vi "FPGA (Top Level) DK.vi"() -> ()   [LabVIEW 2017]
uses:
  <vilib>/LabVIEW Targets/FPGA/cRIO/cRIO-9505/controls.llb/_nicrio_cRIO-9505_DriveStatus.ctl
  <vilib>/Platform/TimedLoop/XDataNode/timing_clust.ctl
  <vilib>/Platform/TimedLoop/XDataNode/nitl_modes.ctl
  <vilib>/Platform/TimedLoop/XDataNode/wakeup.ctl
  <vilib>/rvi/FXPMathLib/FxpSinAndCos/subVIs/nifxpmath_SinAndCos_SimConfig.ctl
  <vilib>/rvi/Emulation/niFpgaGetClockAttributes.vi
  <vilib>/rvi/Emulation/niFpgaSctlEmulationGetInTimedLoop.vi
  <vilib>/rvi/Emulation/niFpgaEmulationReportErrorSimple.vi
  <vilib>/rvi/eio/common/nirviEmuTemplateMethod_errors.vi
  <vilib>/rvi/Emulation/niFpgaEmulationIsFPGAContextNoSignature.vi
  <vilib>/rvi/DataTransferAndStorage/Container/Common/niFpgaContainerGetUniqueNameForEmu.vi
  <vilib>/rvi/Memory/Memory_Emulation/niFpgaMemoryEmulationCacheClearOnFirstRun.vi
  <vilib>/rvi/Memory/Memory_Emulation/nirvimemoryEmulationManagerCache_MakeExclusive.vi
  <vilib>/rvi/Memory/Memory_Emulation/niFpgaMemoryEmulationValidateCache.vi
  <vilib>/rvi/Memory/Memory_Emulation/nirvimemoryEmulationManagerCache_InsertValue.vi
  <vilib>/Utility/error.llb/Clear Errors.vi
  <vilib>/rvi/Memory/Memory_Emulation/nirvimemoryEmulationManagerCache_ReleaseExclusive.vi
  <vilib>/rvi/Memory/Memory_Emulation/nirvimemoryEmulationManagerCache_GetValue.vi
  <vilib>/rvi/Memory/Memory_Emulation/nirvimemoryEmulationManagerCache_SetValue.vi
  <vilib>/rvi/Emulation/niFpgaProcessEmulError.vi
  <vilib>/rvi/Emulation/niFpgaCriticalErrorInLSC.vi
  <vilib>/rvi/FXPMathLib/FxpSinAndCos/simVIs/DllFxpSinAndCosTemp_sub.vi
  <vilib>/eio/EIONode/EIONode.xnode
  <vilib>/rvi/DataTransferAndStorage/Container/XNode/niFpgaContainer.xnode
  <vilib>/rvi/DataTransferAndStorage/Register/Emulation/niFpgaRegisterEmulation.vi
  <vilib>/rvi/FXPMathLib/FxpSinAndCos/XNode/nifxpmath_SinAndCos.xnode
  <vilib>/Platform/TimedLoop/XDataNode/XDataNode.xnode
  <vilib>/Platform/TimedLoop/XDataNode/XDNodeRunTimeDep.lvlib
  <vilib>/eio/EIOMethodNode/EIOMethodNode.xnode
panel:
  in  "Link_1 Duty":i16
  in  "Link_2 Duty":i16
  in  "LINK1_DRIVE_ENABLED":bool
  in  "LINK2_DRIVE_ENABLED":bool
  out "LINK2_DRIVE_STATUS":T1
  out "LINK1_DRIVE_STATUS":T1
  in  "LINK1_LENGTH_MM":fxp<+,16,12>=2.0 format="%#_19g"
  in  "LINK2_LENGTH_MM":fxp<+,16,12>=2.0 format="%#_19g"
  in  "X_OFFSET_MM":fxp<+/-,33,15>
  in  "Y_OFFSET_MM":fxp<+/-,33,15>
  out "LINK2_Y_MM":fxp<+/-,34,16>
  out "LINK2_X_MM":fxp<+/-,34,16>
  out "LINK1_Y_MM":fxp<+/-,34,16>
  out "LINK1_X_MM":fxp<+/-,34,16>
  out "Link 1 Test Y Direction":fxp<+/-,34,16>
  out "LINK1_ENC_POS":i32
  out "LINK2_ENC_POS":i32
  out "LINK1_POT_POS":i32
  out "LINK2_POT_POS":i32
  in  "LINK1_ENC_SCALE":fxp<+,32,0> format="%#_32g"
  in  "LINK2_ENC_SCALE":fxp<+,32,0>=0.029296900611370802 format="%#_32g"
  in  "LINK1_PWM_MAX":i16
  in  "LINK2_PWM_MAX":i16
  in  "LINK1_DEMAND_PWM":i16
  in  "LINK2_DEMAND_PWM":i16
  in  "LINK1_POT_SCALE":fxp<+/-,32,16>
  in  "LINK1_OFFSET":fxp<+/-,16,16>
  in  "LINK2_POT_SCALE":fxp<+/-,32,16>
  in  "LINK2_OFFSET":fxp<+/-,16,16>
  in  "AI_POT_LOOP_US":u16
  in  "ENC_DEBOUNCE_CYCLES":u16=5
  in  "LINK1_ENC_CNTS":i32
  in  "LINK2_ENC_CNTS":i32
  in  "LINK1_UPDATE_ENC":bool
  in  "LINK2_UPDATE_ENC":bool
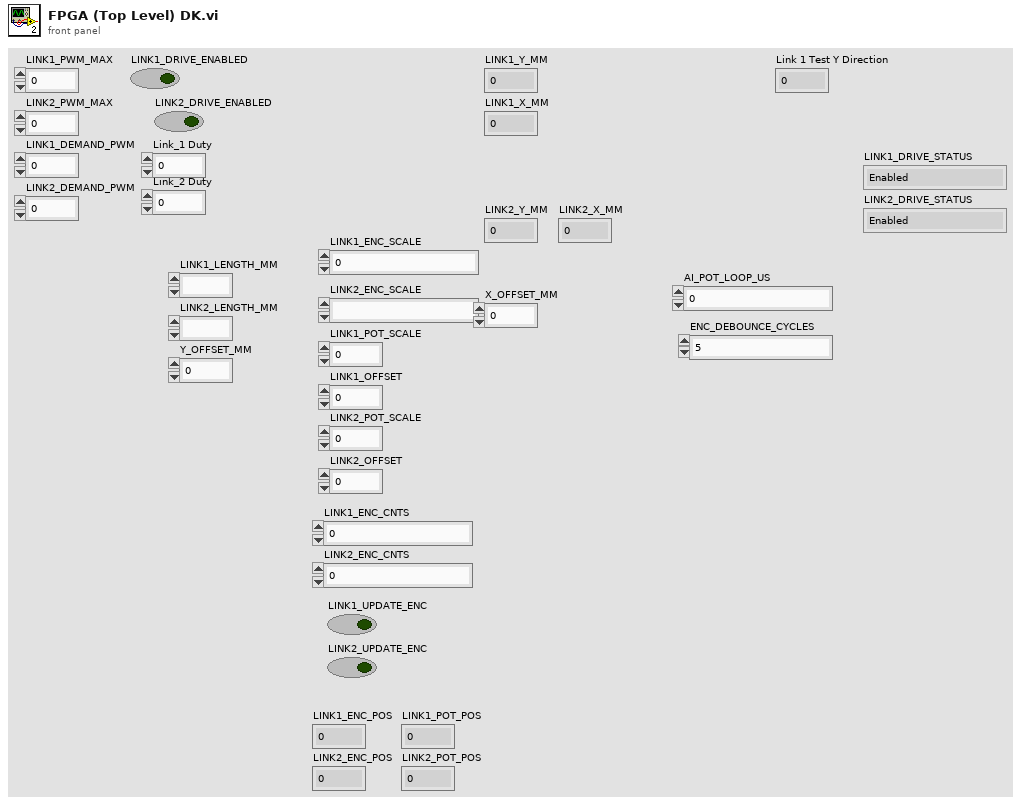
[diagram p1: front panel]
types:
  T1 = typedef "_nicrio_cRIO-9505_DriveStatus.ctl" = enum8{"Enabled", "Disabled", "Disabled by Drive Fault", "Disabled by Temp. Fault", "Disabled by E-Stop", "Unknown"}
  T2 = typedef "XDNodeRunTimeDep.lvlib/timing_clust.ctl" = cluster{"Expected End [f-1]":u64, "Actual End [f-1]":u64, "Finished Late? [f-1]":bool, "Expected End [i-1]":u64, "Actual End [i-1]":u64, "Finished Late? [i-1]":bool, "Expected Start [i]":u64, "Actual Start [i]":u64, "Expected Start [f]":u64, "Actual Start [f]":u64, "Source Name":string, "Structure Name":string, "Period":i64, "Deadline":i64, "Offset":i64, "Start":i64, "Priority":i32, "Timeout":i32, "Mode":T3, "Wakeup Reason":T4, "Error":errorcluster, "Source Type":string, "Secondary Source Type":string, "Global End Time":u64, "Global Start Time":u64, "Frame Duration":u64, "Iteration Duration":u64, "Assigned CPU":i32, "I/O Scan Engine Mode":u32}
  T3 = typedef "XDNodeRunTimeDep.lvlib/nitl_modes.ctl" = enum32{"No Change", "Process missed periods, maintain original phase", "Discard missed periods, maintain original phase", "Process missed periods, ignore original phase", "Discard missed periods, ignore original phase"}
  T4 = typedef "XDNodeRunTimeDep.lvlib/wakeup.ctl" = enum32{"Normal", "Aborted", "Asynchronous wakeup", "Timing source error", "Timed loop error", "Timeout"}
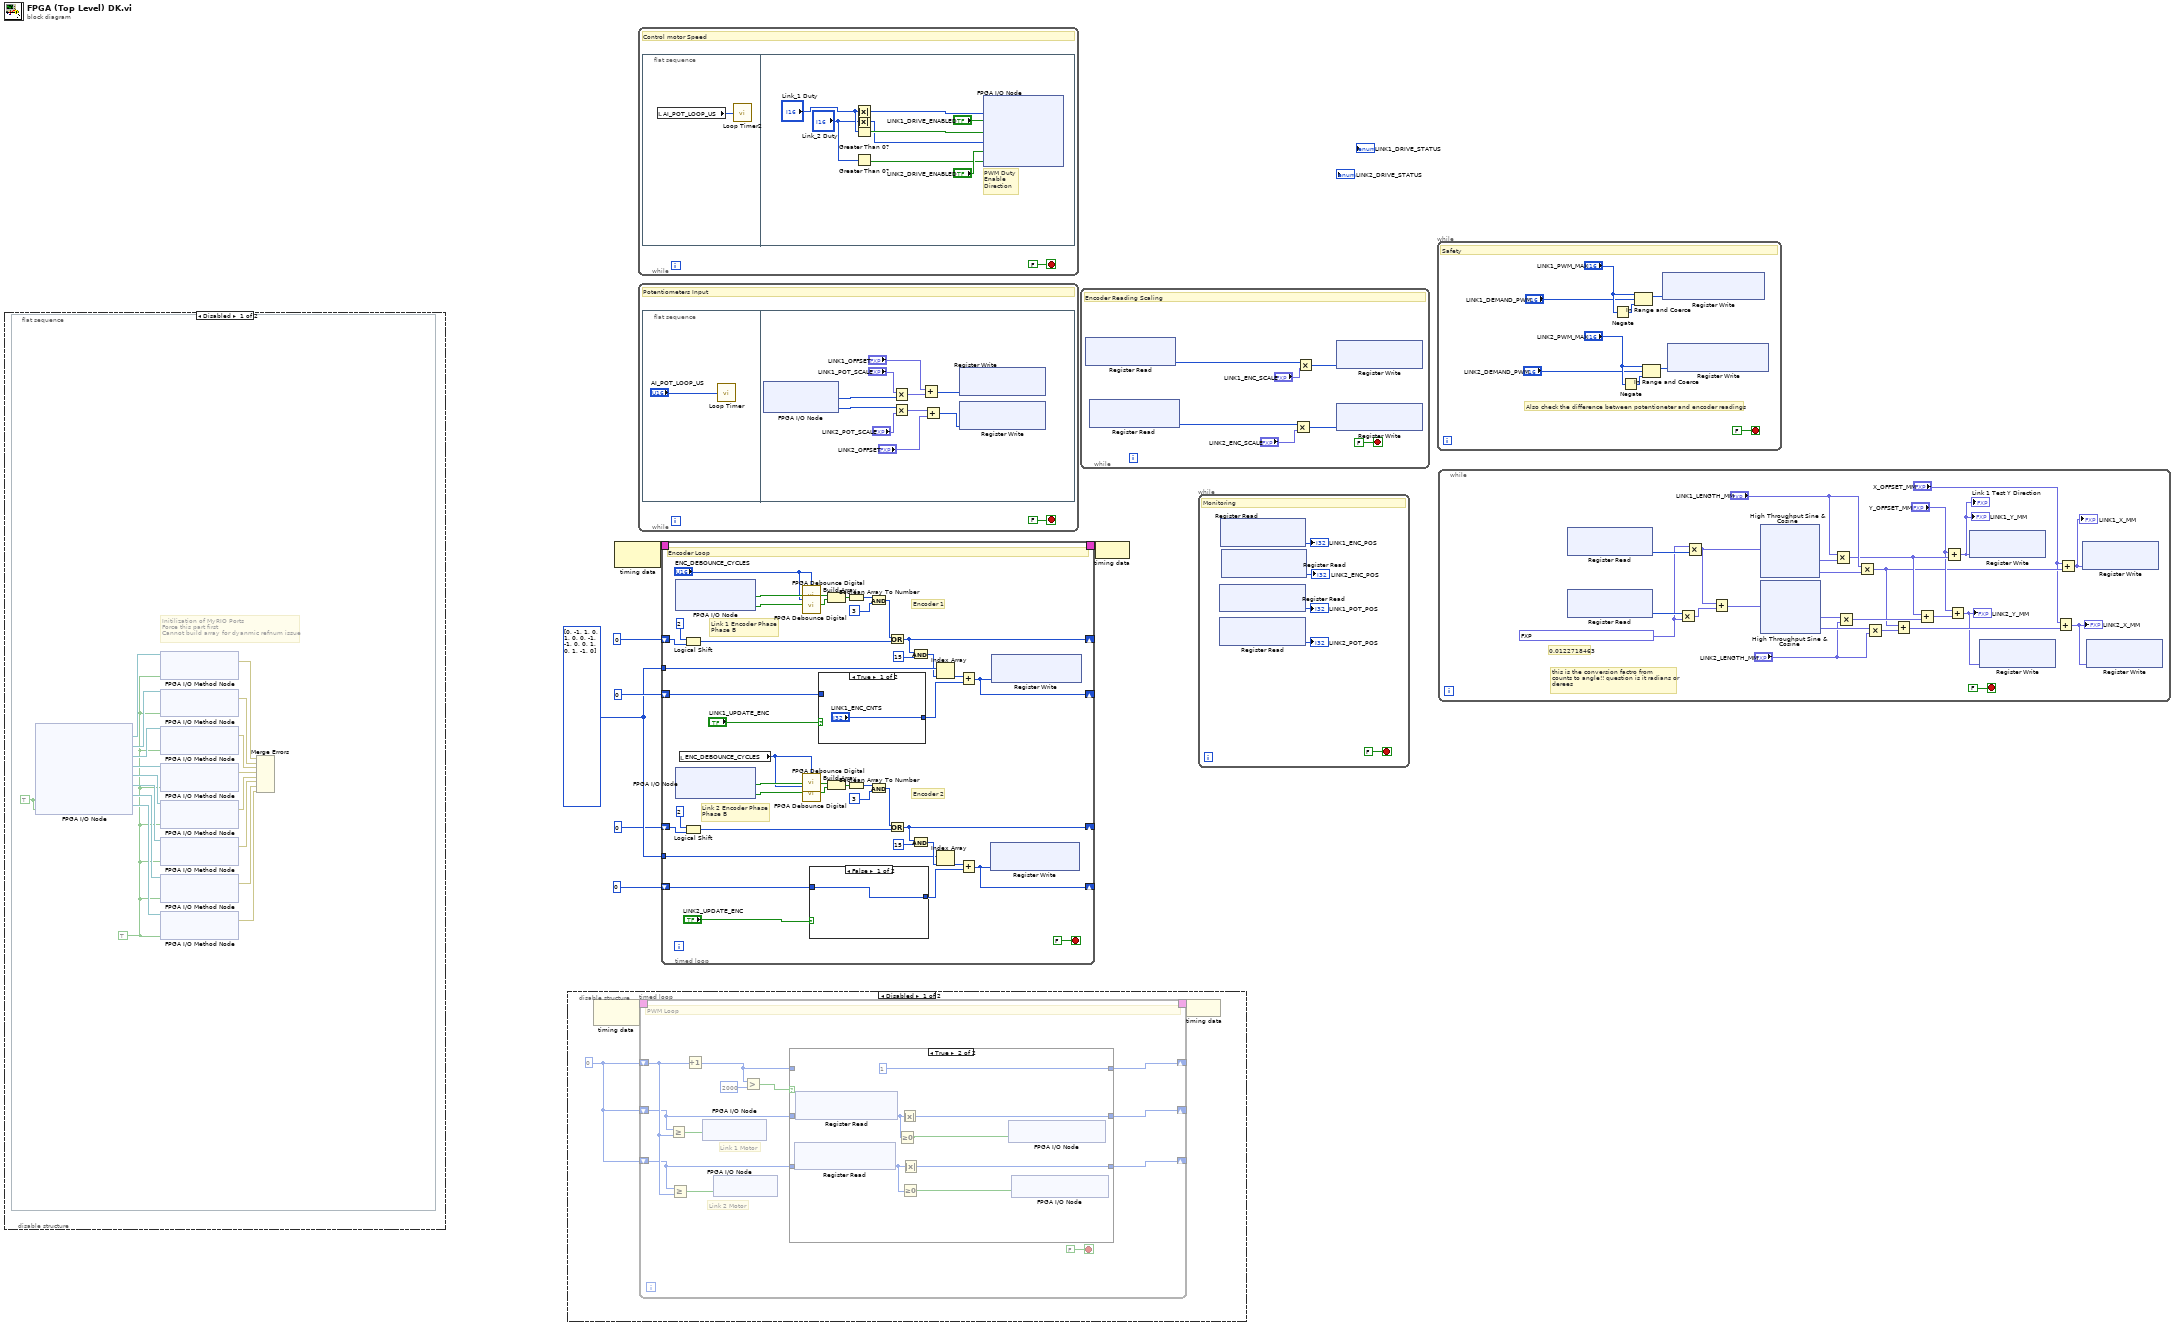
[diagram p0: block diagram]
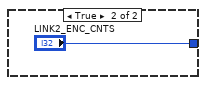
[diagram p5: hidden frame]
diagram:
  w3 = i8[] [0, -1, 1, 0, 1, 0, 0, -1, -1, 0, 0, 1, 0, 1, -1, 0]
  n1 = disable-structure shown="Disabled" {
    frame Disabled {
      n2 = flat-sequence {
        frame #0 {
          w16 = TRUE ("Link 2 Encoder Phase B")
          w25 = TRUE ("Link 2 Encoder Phase B")
          # "Initilization of MyRIO Ports\nForce this part first \nCannot build array for dyanmic refnum issue"
          n3 = xnode "FPGA I/O Node"("Link 2 Encoder Phase B"=w25, "Motor 2 Drive Direction"=w25) -> ("FPGA I/O Out"=w24:refnum<k21>, "FPGA I/O Out"=w23:refnum<k21>, "FPGA I/O Out"=w22:refnum<k21>, "FPGA I/O Out"=w21:refnum<k21>, "FPGA I/O Out"=w20:refnum<k21>, "FPGA I/O Out"=w19:refnum<k21>, "FPGA I/O Out"=w18:refnum<k21>, "FPGA I/O Out"=w17:refnum<k21>)  [unwired: 8 in, 6 out]
          n4 = xnode "FPGA I/O Method Node"("FPGA I/O In"=w24, "Enable"=w16) -> ("error out"=w15:errorcluster)  [unwired: 1 in, 1 out]
          n5 = xnode "FPGA I/O Method Node"("FPGA I/O In"=w23, "Enable"=w16) -> ("error out"=w14:errorcluster)  [unwired: 1 in, 1 out]
          n6 = xnode "FPGA I/O Method Node"("FPGA I/O In"=w22, "Enable"=w16) -> ("error out"=w13:errorcluster)  [unwired: 1 in, 1 out]
          n7 = xnode "FPGA I/O Method Node"("FPGA I/O In"=w21, "Enable"=w16) -> ("error out"=w12:errorcluster)  [unwired: 1 in, 1 out]
          n8 = xnode "FPGA I/O Method Node"("FPGA I/O In"=w20, "Enable"=w16) -> ("error out"=w11:errorcluster)  [unwired: 1 in, 1 out]
          n9 = xnode "FPGA I/O Method Node"("FPGA I/O In"=w19, "Enable"=w16) -> ("error out"=w10:errorcluster)  [unwired: 1 in, 1 out]
          n10 = xnode "FPGA I/O Method Node"("FPGA I/O In"=w18, "Enable"=w16) -> ("error out"=w9:errorcluster)  [unwired: 1 in, 1 out]
          n11 = xnode "FPGA I/O Method Node"("FPGA I/O In"=w17, "Enable"=w16) -> ("error out"=w8:errorcluster)  [unwired: 1 in, 1 out]
          n12 = Merge Errors(w15, w14, w13, w12, w11, w10, w9, w8) -> ()  [unwired: 1 out]
        }
      }
    }
    frame Enabled {
    }
  }
  n13 = disable-structure shown="Disabled" {
    frame Disabled {
      w26 = i16 0 ("Motor 1 PWM Duty Cycle")
      n14 = node-c288() -> (w28:T2)  [unwired: 1 in]
      n15 = timed-loop {
        timing: w28 -> [_]
        timing-out: [_] -> w27
        shift-right: [w39] -> _
        shift-left: w26 -> [w38]
        shift-right: [w37] -> _
        shift-left: w26 -> [w35]
        shift-right: [w36] -> _
        shift-left: w26 -> [w34]
        stop <- FALSE stop-if-true
        # "Link 2 Motor"
        # "Link 1 Motor"
        # "PWM Loop"
        n16 = Greater Or Equal?(x=w35, y=w38) -> (x >= y?=w30:bool)
        n17 = Greater Or Equal?(x=w34, y=w38) -> (x >= y?=w29:bool)
        n18 = Increment(x=w38) -> (x+1=w32:i16)
        n19 = xnode "FPGA I/O Node"("Link 1 Motor"=w30) -> ()  [unwired: 1 in, 1 out]
        n20 = xnode "FPGA I/O Node"("Link 2 Motor"=w29) -> ()  [unwired: 1 in, 1 out]
        n21 = Greater?(x=w32, y=i16 2000) -> (0:w33:bool)
        n22 = case shown="True" w33 {
          tunnel: w32 -> [w43 _]
          tunnel: [w43 i16 1 ("Motor 1 PWM Duty Cycle")] -> w39
          tunnel: [w42 w49] -> w37
          tunnel: [w41 w48] -> w36
          tunnel: w35 -> [w42 _]
          tunnel: w34 -> [w41 _]
          frame False {
          }
          frame True {
            n23 = xnode ("Register Read")() -> ("Data"=w46:i16)  [unwired: 1 in, 1 out]
            n24 = xnode ("Register Read")() -> ("Data"=w47:i16)  [unwired: 1 in, 1 out]
            n25 = Greater Or Equal To 0?(x=w47) -> (x >= 0?=w44:bool)
            n26 = Absolute Value(x=w47) -> (abs(x)=w49:i16)
            n27 = Greater Or Equal To 0?(x=w46) -> (x >= 0?=w45:bool)
            n28 = Absolute Value(x=w46) -> (abs(x)=w48:i16)
            n29 = xnode "FPGA I/O Node"("Motor 1 Drive Direction"=w44) -> ()  [unwired: 1 in, 1 out]
            n30 = xnode "FPGA I/O Node"("Motor 2 Drive Direction"=w45) -> ()  [unwired: 1 in, 1 out]
          }
        }
      }
      n31 = node-c288(w27) -> ()
    }
    frame Enabled {
    }
  }
  n32 = node-c288() -> (w7:T2)  [unwired: 1 in]
  n33 = while {
    stop <- FALSE stop-if-true
    # "Control motor Speed"
    n34 = flat-sequence {
      frame #0 {
        n35 = local read "AI_POT_LOOP_US"() -> (w56:u16)
        n36 = call "Loop Timer2"("Count(uSec)"=w56) -> ()  [unwired: 1 out]
      }
      frame #1 {
        # "PWM Duty\nEnable\nDirection"
        n37 = Absolute Value(x="Link_1 Duty") -> (abs(x)=w57:i16)
        n38 = Absolute Value(x="Link_2 Duty") -> (abs(x)=w58:i16)
        n39 = Greater Than 0?(x="Link_1 Duty") -> (x > 0?=w59:bool)
        n40 = Greater Than 0?(x="Link_2 Duty") -> (x > 0?=w60:bool)
        n41 = xnode "FPGA I/O Node"("ConnectorC/AO0"=w57, "ConnectorC/DIO0"="LINK1_DRIVE_ENABLED", "ConnectorC/DIO1"=w59, "ConnectorC/AO1"=w58, "ConnectorC/DIO2"="LINK2_DRIVE_ENABLED", "ConnectorC/DIO3"=w60) -> ()  [unwired: 6 in, 6 out]
      }
    }
  }
  n42 = while {
    stop <- FALSE stop-if-true
    # "Potentiometers Input"
    n43 = flat-sequence {
      frame #0 {
        n44 = call "Loop Timer"("Count(uSec)"="AI_POT_LOOP_US") -> ()  [unwired: 1 out]
      }
      frame #1 {
        n45 = xnode "FPGA I/O Node"() -> ("ConnectorB/AI1"=w68:u16, "ConnectorB/AI2"=w67:u16)  [unwired: 2 in, 2 out]
        n46 = Multiply(x="LINK1_POT_SCALE", y=w68) -> (x*y=w75:fxp<+/-,48,32>)
        n47 = Multiply(x=w67, y="LINK2_POT_SCALE") -> (x*y=w71:fxp<+/-,48,32>)
        n48 = Add(x="LINK1_OFFSET", y=w75) -> (x+y=w69:i32)
        n49 = Add(x=w71, y="LINK2_OFFSET") -> (x+y=w70:i32)
        n50 = xnode ("Register Write")("Data"=w69) -> ()  [unwired: 1 in, 1 out]
        n51 = xnode ("Register Write")("Data"=w70) -> ()  [unwired: 1 in, 1 out]
      }
    }
  }
  n52 = timed-loop {
    timing: w7 -> [_]
    timing-out: [_] -> w6
    tunnel: w3 -> [w116]
    shift-right: [w109] -> _
    shift-left: u8 0 -> [w118]
    shift-right: [w80] -> _
    shift-left: 0 -> [w101]
    tunnel: w3 -> [w85]
    shift-right: [w83] -> _
    shift-left: u8 0 -> [w84]
    shift-right: [w79] -> _
    shift-left: 0 -> [w77]
    stop <- FALSE stop-if-true
    # "Link 2 Encoder Phase \nPhase B"
    # "Link 1 Encoder Phase \nPhase B"
    # "Encoder 2"
    # "Encoder 1"
    # "Encoder Loop"
    n53 = xnode "FPGA I/O Node"() -> ("ConnectorC/DIO4"=w107:bool, "ConnectorC/DIO5"=w106:bool)  [unwired: 2 in, 2 out]
    n54 = xnode "FPGA I/O Node"() -> ("ConnectorC/DIO6"=w91:bool, "ConnectorC/DIO7"=w90:bool)  [unwired: 2 in, 2 out]
    n55 = local read "ENC_DEBOUNCE_CYCLES"() -> (w82:u16)
    n56 = Logical Shift(y=i16 2, x=w118) -> (x << y=w111:u8)
    n57 = Logical Shift(y=i16 2, x=w84) -> (x << y=w94:u8)
    n58 = call "FPGA Debounce Digital.vi"("Input Signal"=w107, "Cycles to Filter"="ENC_DEBOUNCE_CYCLES") -> ("Output Filtered Signal"=w105:bool)
    n59 = call "FPGA Debounce Digital.vi"("Input Signal"=w106, "Cycles to Filter"="ENC_DEBOUNCE_CYCLES") -> ("Output Filtered Signal"=w104:bool)
    n60 = call "FPGA Debounce Digital.vi"("Input Signal"=w91, "Cycles to Filter"=w82) -> ("Output Filtered Signal"=w89:bool)
    n61 = call "FPGA Debounce Digital.vi"("Input Signal"=w90, "Cycles to Filter"=w82) -> ("Output Filtered Signal"=w88:bool)
    n62 = case shown="False" "LINK2_UPDATE_ENC" {
      tunnel: w77 -> [w120 _]
      tunnel: [w120 "LINK2_ENC_CNTS"] -> w86
      frame False {
      }
      frame True {
      }
    }
    n63 = case shown="True" "LINK1_UPDATE_ENC" {
      tunnel: w101 -> [_ w123]
      tunnel: ["LINK1_ENC_CNTS" w123] -> w100
      frame True {
      }
      frame False {
      }
    }
    n64 = Build Array(w105, w104) -> (w103:bool[])
    n65 = Build Array(w89, w88) -> (w87:bool[])
    n66 = Boolean Array To Number(Boolean array=w103) -> (number=w114:u8)
    n67 = Boolean Array To Number(Boolean array=w87) -> (number=w97:u8)
    n68 = And(x=w114, y=u8 3) -> (x .and. y?=w112:u8)
    n69 = And(x=w97, y=u8 3) -> (x .and. y?=w95:u8)
    n70 = Or(x=w112, y=w111) -> (x .or. y?=w109:u8)
    n71 = Or(x=w95, y=w94) -> (x .or. y?=w83:u8)
    n72 = And(x=w109, y=u8 15) -> (x .and. y?=w110:u8)
    n73 = And(x=w83, y=u8 15) -> (x .and. y?=w93:u8)
    n74 = Index Array(array=w116, index=w110) -> (element=w108:i8)
    n75 = Index Array(array=w85, index=w93) -> (element=w92:i8)
    n76 = Add(x=w108, y=w100) -> (x+y=w80:i32)
    n77 = Add(x=w92, y=w86) -> (x+y=w79:i32)
    n78 = xnode ("Register Write")("Data"=w79) -> ()  [unwired: 1 in, 1 out]
    n79 = xnode ("Register Write")("Data"=w80) -> ()  [unwired: 1 in, 1 out]
  }
  n80 = while {
    stop <- FALSE stop-if-true
    # "Encoder Reading Scaling"
    n81 = xnode ("Register Read")() -> ("Data"=w130:i32)  [unwired: 1 in, 1 out]
    n82 = xnode ("Register Read")() -> ("Data"=w131:i32)  [unwired: 1 in, 1 out]
    n83 = Multiply(x=w131, y="LINK2_ENC_SCALE") -> (x*y=w128:i32)
    n84 = Multiply(x=w130, y="LINK1_ENC_SCALE") -> (x*y=w129:i32)
    n85 = xnode ("Register Write")("Data"=w129) -> ()  [unwired: 1 in, 1 out]
    n86 = xnode ("Register Write")("Data"=w128) -> ()  [unwired: 1 in, 1 out]
  }
  n87 = node-c288(w6) -> ()
  n88 = while {
    stop <- FALSE stop-if-true
    # "Monitoring"
    n89 = xnode ("Register Read")() -> ("Data"=→"LINK1_POT_POS":i32)  [unwired: 1 in, 1 out]
    n90 = xnode ("Register Read")() -> ("Data"=→"LINK2_POT_POS":i16)  [unwired: 1 in, 1 out]
    n91 = xnode ("Register Read")() -> ("Data"=→"LINK1_ENC_POS":i32)  [unwired: 1 in, 1 out]
    n92 = xnode ("Register Read")() -> ("Data"=→"LINK2_ENC_POS":i32)  [unwired: 1 in, 1 out]
  }
  n93 = while {
    stop <- FALSE stop-if-true
    # "Also check the difference between potentioneter and encoder readings"
    # "Safety"
    n94 = Negate(x="LINK1_PWM_MAX") -> (-x=w144:i16)
    n95 = Negate(x="LINK2_PWM_MAX") -> (-x=w142:i16)
    n96 = In Range and Coerce(upper limit="LINK1_PWM_MAX", x="LINK1_DEMAND_PWM", lower limit=w144) -> (coerced(x)=w145:i16)  [unwired: 1 out]
    n97 = In Range and Coerce(upper limit="LINK2_PWM_MAX", x="LINK2_DEMAND_PWM", lower limit=w142) -> (coerced(x)=w141:i16)  [unwired: 1 out]
    n98 = xnode ("Register Write")("Data"=w145) -> ()  [unwired: 1 in, 1 out]
    n99 = xnode ("Register Write")("Data"=w141) -> ()  [unwired: 1 in, 1 out]
  }
  n100 = while {
    stop <- FALSE stop-if-true
    w147 = fxp<+,31,-8> 5.555555617320351e-05
    # "0.0122718463"
    # "this is the conversion factro from \ncounts to angle!! question is it radians or\nderees"
    n101 = xnode ("Register Read")() -> ("Data"=w153:i32)  [unwired: 1 in, 1 out]
    n102 = xnode ("Register Read")() -> ("Data"=w170:i32)  [unwired: 1 in, 1 out]
    n103 = Multiply(x=w170, y=w147) -> (x*y=w169:fxp<+/-,63,24>)
    n104 = Multiply(x=w147, y=w153) -> (x*y=w152:fxp<+/-,63,24>)
    n105 = Add(x=w152, y=w169) -> (x+y=w168:fxp<+/-,64,25>)
    n106 = xnode "High Throughput Sine & Cosine"("x (pi)"=w152) -> ("sin(x)"=w167:fxp<+/-,16,2>, "cos(x)"=w166:fxp<+/-,16,2>)
    n107 = xnode "High Throughput Sine & Cosine"("x (pi)"=w168) -> ("sin(x)"=w164:fxp<+/-,16,2>, "cos(x)"=w163:fxp<+/-,16,2>)
    n108 = Multiply(x="LINK1_LENGTH_MM", y=w167) -> (x*y=w159:fxp<+/-,32,14>)
    n109 = Multiply(x=w164, y="LINK2_LENGTH_MM") -> (x*y=w160:fxp<+/-,32,14>)
    n110 = Multiply(x="LINK1_LENGTH_MM", y=w166) -> (x*y=w156:fxp<+/-,32,14>)
    n111 = Multiply(x=w163, y="LINK2_LENGTH_MM") -> (x*y=w161:fxp<+/-,32,14>)
    n112 = Add(x=w156, y=w161) -> (x+y=w155:fxp<+/-,33,15>)
    n113 = Add(x=w159, y=w160) -> (x+y=w158:fxp<+/-,33,15>)
    n114 = Add(x="Y_OFFSET_MM", y=w159) -> (x+y=w149:fxp<+/-,34,16>)
    "LINK1_Y_MM" <- w149
    "Link 1 Test Y Direction" <- w149
    n115 = Add(x="Y_OFFSET_MM", y=w158) -> (x+y=w151:fxp<+/-,34,16>)
    "LINK2_Y_MM" <- w151
    n116 = xnode ("Register Write")("Data"=w149) -> ()  [unwired: 1 in, 1 out]
    n117 = xnode ("Register Write")("Data"=w151) -> ()  [unwired: 1 in, 1 out]
    n118 = Add(x="X_OFFSET_MM", y=w155) -> (x+y=w150:fxp<+/-,34,16>)
    "LINK2_X_MM" <- w150
    n119 = Add(x="X_OFFSET_MM", y=w156) -> (x+y=w148:fxp<+/-,34,16>)
    "LINK1_X_MM" <- w148
    n120 = xnode ("Register Write")("Data"=w148) -> ()  [unwired: 1 in, 1 out]
    n121 = xnode ("Register Write")("Data"=w150) -> ()  [unwired: 1 in, 1 out]
  }
